vi "FindServerByName.vi"(0 "Servers":T1[](array[typedef]), 5 "Name":string) -> (4 "Found":bool, 6 "Index":i32)   [LabVIEW 2020]
uses:
  <vilib>/WebServerConfig/Server.ctl
  <vilib>/WebServerConfig/Alias.ctl
  <vilib>/WebServerConfig/ErrorDocument.ctl
  <vilib>/WebServerConfig/Action.ctl
  <vilib>/WebServerConfig/Redirect.ctl
  <vilib>/WebServerConfig/Interface.ctl
  <vilib>/WebServerConfig/AddHandler.ctl
  <vilib>/WebServerConfig/SSL.ctl
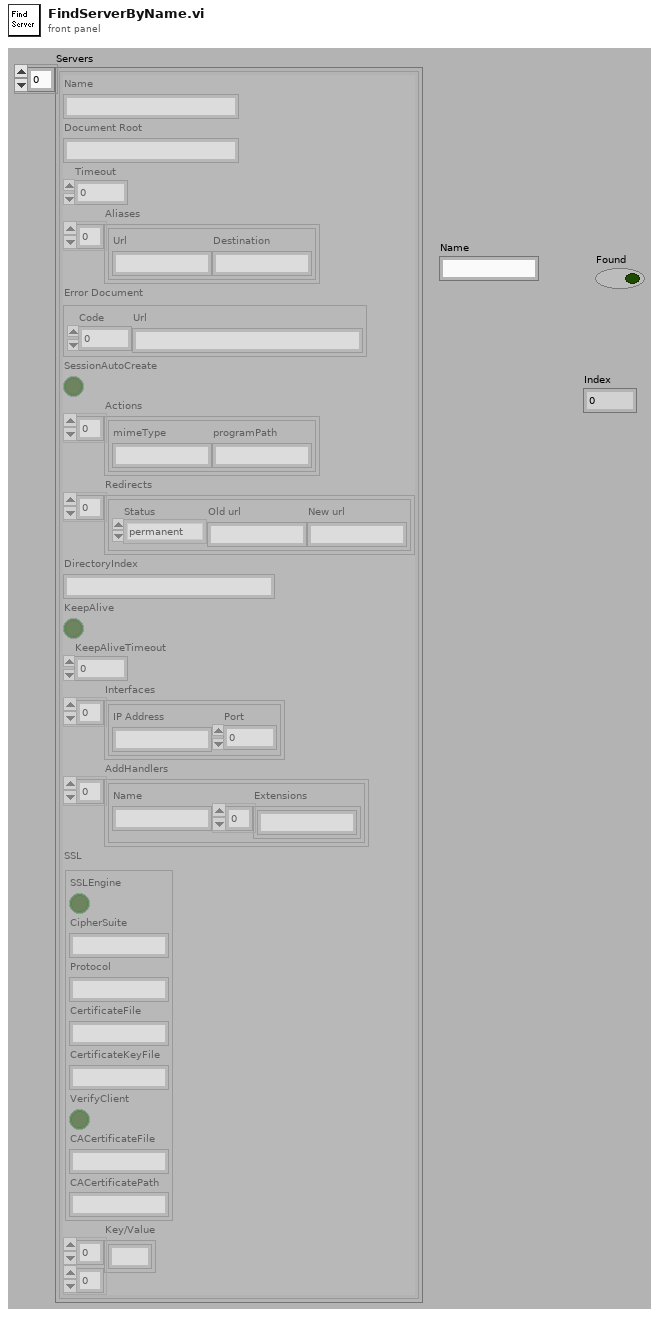
[diagram p1: front panel]
types:
  T1 = typedef "Server.ctl" = cluster{"Name":string, "Document Root":string, "Timeout":u32, "Aliases":T2[], "Error Document":T3, "SessionAutoCreate":bool, "Actions":T4[], "Redirects":T5[], "DirectoryIndex":string, "KeepAlive":bool, "KeepAliveTimeout":u32, "Interfaces":T6[], "AddHandlers":T7[], "SSL":T8, "Key/Value":string[][]}
  T2 = typedef "Alias.ctl" = cluster{"Url":string, "Destination":string}
  T3 = typedef "ErrorDocument.ctl" = cluster{"Code":u16, "Url":string}
  T4 = typedef "Action.ctl" = cluster{"mimeType":string, "programPath":string}
  T5 = typedef "Redirect.ctl" = cluster{"Status":enum16{"permanent", "temp", "seeother", "gone"}, "Old url":string, "New url":string}
  T6 = typedef "Interface.ctl" = cluster{"IP Address":string, "Port":u16}
  T7 = typedef "AddHandler.ctl" = cluster{"Name":string, "Extensions":string[]}
  T8 = typedef "SSL.ctl" = cluster{"SSLEngine":bool, "CipherSuite":string, "Protocol":string, "CertificateFile":string, "CertificateKeyFile":string, "VerifyClient":bool, "CACertificateFile":string, "CACertificatePath":string}
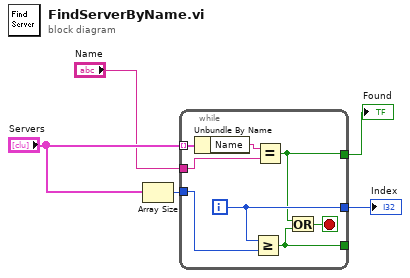
[diagram p0: block diagram]
diagram:
  n1 = Array Size(array="Servers") -> (size(s)=w2:i32)
  n2 = while {
    tunnel: "Servers" -> [w13] mode=indexing
    tunnel: "Name" -> [w7]
    tunnel: w2 -> [w12]
    tunnel: [w10] -> w4
    tunnel: [w9] -> _
    tunnel: [w8] -> w3
    i -> [w10]
    stop <- w6 stop-if-true
    n3 = Unbundle By Name(w13) -> ("Name"=w11:string)
    n4 = Greater Or Equal?(x=w10, y=w12) -> (x >= y?=w9:bool)
    n5 = Equal?(x=w11, y=w7) -> (x = y?=w8:bool)
    n6 = Or(x=w8, y=w9) -> (x .or. y?=w6:bool)
  }
  "Index" <- w4
  "Found" <- w3
